vi "Build Basic Bus Monitor.vi"(6 "48-bit Time Tag":bool, 8 "error in (no error)":errorcluster, 11 "Bus Monitor in":refnum<class "Bus Monitor.lvclass">) -> (0 "error out":errorcluster, 3 "Bus Monitor out":refnum<class "Bus Monitor.lvclass">)   [LabVIEW 2020, in "Unit Tests.lvlib" / "Bus Monitor.lvclass"]
uses:
  Bus Monitor.lvclass
  Bus Monitor/TypeDefs/Bus Monitor Configuration.ctl
  Bus Monitor/TypeDefs/Bus Monitor Timeout.ctl
  Bus Monitor/TypeDefs/Bus Monitor Timetag Behavior.ctl
  Bus Monitor/TypeDefs/Bus Monitor Record Requirement.ctl
  Bus Monitor/TypeDefs/Bus Monitor Timetag Configuration.ctl
  Filters/TypeDefs/Filter Configuration.ctl
  Frames & Messages/TypeDefs/Command Type.ctl
  Frames & Messages/TypeDefs/Command Terminal Address.ctl
  Frames & Messages/TypeDefs/Command SubAddress.ctl
  Frames & Messages/TypeDefs/Simplified Parameter Data Table.ctl
  Frames & Messages/TypeDefs/Scaling Information.ctl
  Bus Monitor.lvclass/Bus Monitor.ctl
  Bus Monitor/Bus Monitor.lvclass
  C:/Users/MattJ/Desktop/git/bci-1553-labview-api/src/1553 SubComponent/1553 SubComponent.lvclass
  1553 Session/1553 Session.lvclass
  Filters/Filter/Filter.lvclass
  BCI-1553 API.lvlib
  1553 Component/1553 Component.lvclass
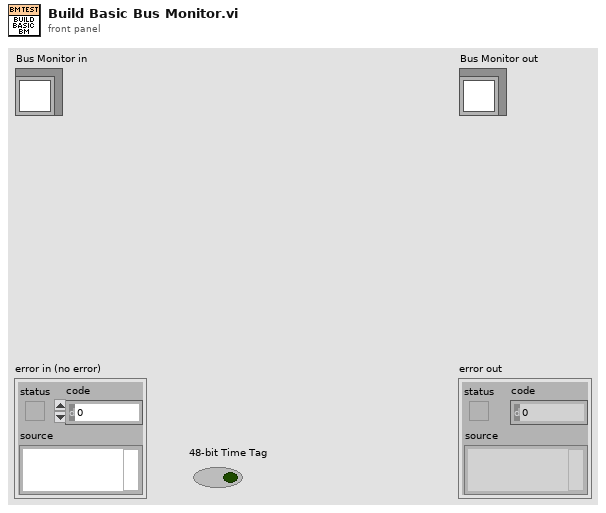
[diagram p1: front panel]
types:
  T1 = typedef "BCI-1553 API.lvlib/Bus Monitor.lvclass/Bus Monitor Record Requirement.ctl" = enum16{"Properly Encoded - Complete - Cmd Sync", "Properly Encoded - Complete - Cmd or Data Sync", "Properly Encoded Cmd Sync - At Least 2 Data Bits ", "Any Properly Encoded Sync - At Least 2 Data Bits"}
  T2 = typedef "BCI-1553 API.lvlib/Bus Monitor.lvclass/Bus Monitor Timetag Behavior.ctl" = enum16{"Last Bit of Last Word", "First Bit of Command Word", "Last Bit of Command Word", "Timetag Disabled"}
  T3 = typedef "BCI-1553 API.lvlib/Bus Monitor.lvclass/Bus Monitor Timeout.ctl" = enum16{"18us", "23us", "82us", "140us"}
  T4 = typedef "BCI-1553 API.lvlib/Simplified Parameter Data Table.ctl" = cluster{"Parameter Name":string, "Base Word":u16, "Scaling Info":T5}
  T5 = typedef "BCI-1553 API.lvlib/Scaling Information.ctl" = cluster{"Bit Offset":i32, "Bit Count":i32, "LSB Resolution":dbl, "2's Complement":bool, "Big Endian":bool, "Sign Bit":bool}
  T6 = typedef "BCI-1553 API.lvlib/Filter Configuration.ctl" = cluster{"Filter Type":T7, "Terminal Address (0-30)":T8, "SubAddress (1-30)":T9, "Mode Code":bool, "Broadcast":bool, "RT-RT":bool, "Bus A":bool}
  T7 = typedef "BCI-1553 API.lvlib/Command Type.ctl" = enum16{"Transmit", "Receive"}
  T8 = typedef "BCI-1553 API.lvlib/Command Terminal Address.ctl" = enum16{"0", "1", "2", "3", "4", "5", "6", "7", "8", "9", "10", "11", "12", "13", "14", "15", "16", "17", "18", "19", "20", "21", "22", "23", "24", "25", "26", "27", "28", "29", "30", "Broadcast"}
  T9 = typedef "BCI-1553 API.lvlib/Command SubAddress.ctl" = enum16{"Mode Code", "1", "2", "3", "4", "5", "6", "7", "8", "9", "10", "11", "12", "13", "14", "15", "16", "17", "18", "19", "20", "21", "22", "23", "24", "25", "26", "27", "28", "29", "30"}
  T10 = typedef "BCI-1553 API.lvlib/Bus Monitor.lvclass/Bus Monitor Configuration.ctl" = cluster{"Timeout":T3, "Gap Check":bool, "Timetag Behavior":T2, "Record Requirement":T1, "Cont Record After Inv Word":bool, "Ext Msg Flag Enable":bool, "48-bit Time Tag":bool, "Simple Mode":bool, "Bus Monitor Timetag Config":T11}
  T11 = typedef "BCI-1553 API.lvlib/Bus Monitor.lvclass/Bus Monitor Timetag Configuration.ctl" = enum16{"Disabled", "2us", "4us", "8us", "16us", "32us", "64us", "100ns"}
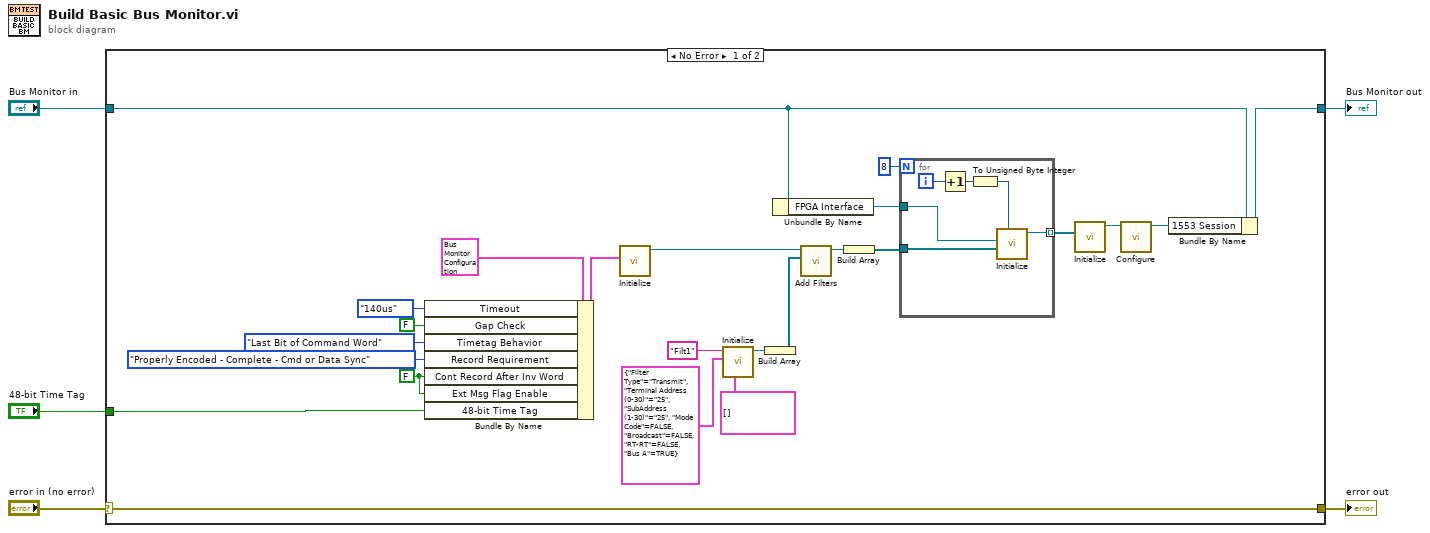
[diagram p0: block diagram]
diagram:
  n1 = case shown="No Error" "error in (no error)" {
    selector: "error in (no error)" -> [w29 w37]
    tunnel: [w29 w37] -> w4
    tunnel: [w8 w36] -> w2
    tunnel: "Bus Monitor in" -> [w9 w36]
    tunnel: "48-bit Time Tag" -> [w18 _]
    frame No Error {
      w26 = FALSE ("Cont Record After Inv Word")
      n2 = Bundle By Name(cluster=T10 {"Timeout"=enum."18us", "Gap Check"=FALSE, "Timetag Behavior"=enum."Last Bit of Last Word", "Record Requirement"=enum."Properly Encoded - Complete - Cmd Sync", "Cont Record After Inv Word"=FALSE, "Ext Msg Flag Enable"=FALSE, "48-bit Time Tag"=FALSE, "Simple Mode"=FALSE, "Bus Monitor Timetag Config"=enum."Disabled"} ("Bus Monitor Configuration"), "Timeout"=Bus_Monitor_Timeout."140us", "Gap Check"=FALSE, "Timetag Behavior"=Bus_Monitor_Timetag_Behavior."Last Bit of Command Word", "Record Requirement"=Bus_Monitor_Record_Requirement."Properly Encoded - Complete - Cmd or Data Sync", "Cont Record After Inv Word"=w26, "Ext Msg Flag Enable"=w26, "48-bit Time Tag"=w18) -> (w27:T10)
      n3 = call "Initialize.vi"("Bus Monitor Configuration"=w27) -> ("Bus Monitor out"=w24:refnum<class "Bus Monitor.lvclass">)  [unwired: 9 in, 1 out]
      n4 = call "Initialize.vi"("Parameters"=T4[] [], "Filter Configuration"=T6 {"Filter Type"=enum."Transmit", "Terminal Address (0-30)"=enum."25", "SubAddress (1-30)"=enum."25", "Mode Code"=FALSE, "Broadcast"=FALSE, "RT-RT"=FALSE, "Bus A"=TRUE}, "ID"="Filt1") -> ("Filter out"=w23:refnum<class "Filter.lvclass">)  [unwired: 7 in, 1 out]
      n5 = Build Array(w23) -> (w22:refnum<class "Filter.lvclass">[])
      n6 = Unbundle By Name(w9) -> ("FPGA Interface"=w14:refnum<class "FPGA Interface.lvclass">)
      n7 = call-dynamic "Add Filters.vi"("Filters"=w22, "Bus Monitor in"=w24) -> ("Bus Monitor out"=w12:refnum<class "Bus Monitor.lvclass">)  [unwired: 8 in, 1 out]
      n8 = Build Array(w12) -> (w13:refnum<class "Bus Monitor.lvclass">[])
      n9 = for {
        N: 8 -> [_]
        tunnel: [w33] -> w10 mode=indexing
        tunnel: w13 -> [w32]
        tunnel: w14 -> [w31]
        i -> [w35]
        n10 = Increment(x=w35) -> (x+1=w30:i32)
        n11 = To Unsigned Byte Integer(number=w30) -> (unsigned 8bit integer=w34:u8)
        n12 = call "Initialize.vi"("Component ID (1-8)"=w34, "SubComponents"=w32, "FPGA Interface"=w31) -> ("1553 Component out"=w33:refnum<class "1553 Component.lvclass">)  [unwired: 7 in, 1 out]
      }
      n13 = call "Initialize.vi"("Components"=w10) -> ("1553 Board out"=w7:refnum<class "1553 Session.lvclass">)  [unwired: 9 in, 1 out]
      n14 = call-dynamic "Configure.vi"("1553 Board in"=w7) -> ("1553 Board out"=w6:refnum<class "1553 Session.lvclass">)  [unwired: 9 in, 1 out]
      n15 = Bundle By Name(cluster=w9, "1553 Session"=w6) -> (w8:refnum<class "Bus Monitor.lvclass">)
    }
    frame Error {
    }
  }
  "error out" <- w4
  "Bus Monitor out" <- w2
